vi "Configure Sys (To) Period.vi"(8 "error in (no error)":errorcluster, 9 "Period (100 msec)":dbl=0.1 format="%.6p", 11 "VISA resource name":refnum<visa-resource-name>) -> (0 "error out":errorcluster, 3 "VISA resource name out":refnum<visa-resource-name>)   [LabVIEW 2013, in "Berkeley Nucleonics 500 Series.lvlib"]
doc: "This VI is used to set the base timer (i.e. System (To)) period.\n\nValid Range: 2.0E-7 to 5000 sec"
uses:
  Berkeley Nucleonics 500 Series.lvlib
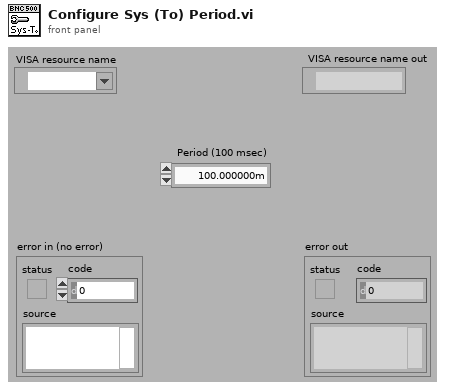
[diagram p1: front panel]
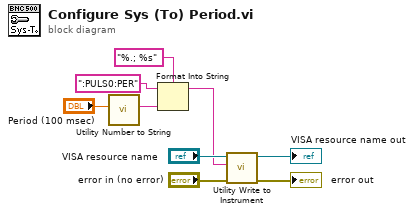
[diagram p0: block diagram]
diagram:
  n1 = call "Utility Number to String.vi"("Numeric"="Period (100 msec)") -> ("Shortest String"=w3:string)  [unwired: 10 in]
  n2 = Format Into String(format string="%.; %s", initial string=":PULS0:PER", w3) -> (resulting string=w1:string)  [unwired: 1 in, 1 out]
  n3 = call "Utility Write to Instrument.vi"("error in (no error)"="error in (no error)", "Write Buffer"=w1, "VISA resource name"="VISA resource name") -> ("error out"=→"error out":errorcluster, "VISA resource name out"=→"VISA resource name out":refnum<visa-resource-name>)  [unwired: 6 in, 1 out]
